vi "validate.vi"(8 "error in":errorcluster, 11 "configuration in":refnum<class "PL_System Configuration.lvclass">) -> (0 "error out":errorcluster, 3 "configuration out":refnum<class "PL_System Configuration.lvclass">)   [LabVIEW 2013, in "PL_System Configuration.lvclass"]
doc: "Provides an interface for performing validation on a given configuration. Any children should define the behavior of this function to ensure that the configuration in memory can be used by the runtime class."
uses:
  PL_System Configuration.lvclass
  <vilib>/NI/Tag Bus Module Framework/root configuration/TBM configuration.lvclass
  PL_System Configuration.lvclass/PL_System Configuration.ctl
  <vilib>/NI/CEF/CEF_TreeControl/NISE_CEF_TreeControl.lvlib
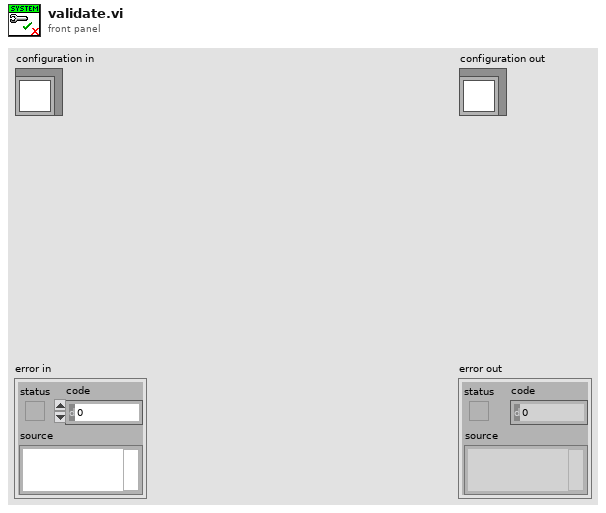
[diagram p1: front panel]
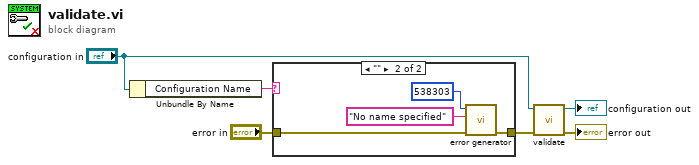
[diagram p0: block diagram]
diagram:
  n1 = Unbundle By Name("configuration in") -> ("Configuration Name"=w1:string)
  n2 = case shown="\"\"" w1 {
    tunnel: [w7 w10] -> w4
    tunnel: "error in" -> [w7 w11]
    frame Default {
    }
    frame "" {
      n3 = call <vilib>:"error generator.vi"("error in"=w11, "append error message"="No name specified" ("error message (\"\")"), "error code (0)"=538303) -> ("error out"=w10:errorcluster)  [unwired: 6 in]
    }
  }
  n4 = call-parent "validate.vi"("error in"=w4, "configuration in"="configuration in") -> ("error out"=→"error out":errorcluster, "configuration out"=→"configuration out":refnum<class "PL_System Configuration.lvclass">)  [unwired: 8 in]
